vi "vew -- array interpolate.vi"() -> ()   [LabVIEW 2010]
uses:
  Q -- check range -- i -- real.vi
  Q - not nan -- real.vi
  <vilib>/gmath/function.llb/Binomial Coefficient.vi
panel:
  in  "N":i32=100
  in  "freq max":dbl=300.0
  in  "freq min":dbl=10.0
  out "Plot: phase around center":cluster{dbl[], dbl[]}[](graph)=[{array[1389 elements], array[1389 elements]}, {[3015.8552146531347, 3016.2383756063605, 3016.6215365595863], [1.7830935388456814, 3.353889865640578, 4.924686192435475]}, {array[1389 elements], array[1389 elements]}]
  in  "all Voltage":dbl[](array[numeric])=[0.1, 0.5, 0.2, 0.9]
  in  "all tempearure":dbl[](array[numeric])=[10.0, 70.0, 150.0, 300.0]
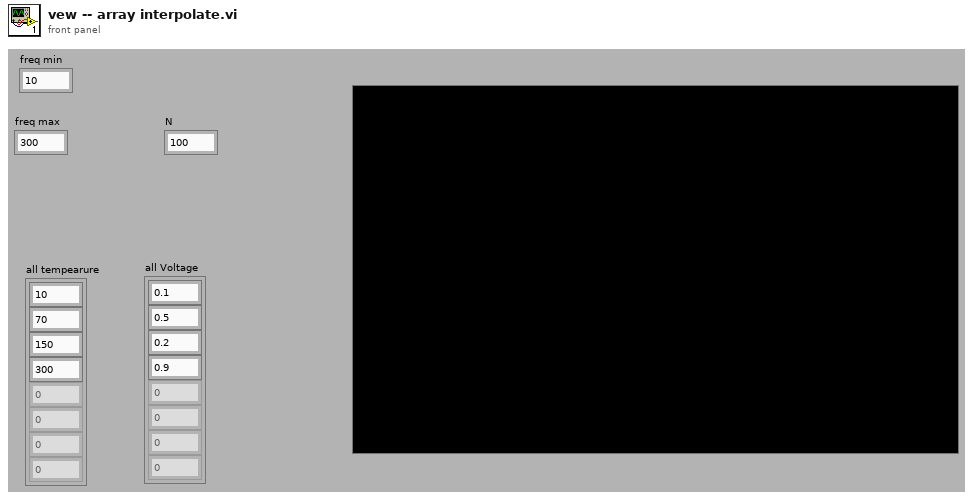
[diagram p1: front panel]
types:
  T1 = cluster{"all tempearure":dbl[], "all Voltage":dbl[]}
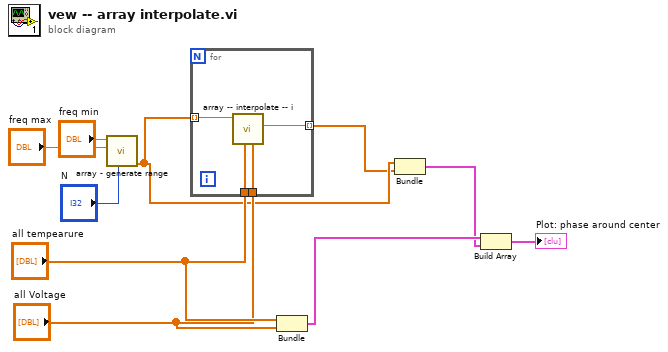
[diagram p0: block diagram]
diagram:
  n1 = call "array - generate range.vi"("N"="N", "freq max"="freq max", "freq min"="freq min") -> ("Array"=w4:dbl[])  [unwired: 8 in]
  n2 = for {
    tunnel: "all tempearure" -> [w14]
    tunnel: "all Voltage" -> [w13]
    tunnel: w4 -> [w12] mode=indexing
    tunnel: [w11] -> w3 mode=indexing
    n3 = call "array -- interpolate -- i.vi"("all Voltage"=w13, "all tempearure"=w14, "temperature (K)"=w12) -> ("V out"=w11:dbl)  [unwired: 8 in]
  }
  n4 = Bundle("all tempearure"="all tempearure", "all Voltage"="all Voltage") -> (w8:T1)  [unwired: 1 in]
  n5 = Bundle("Array"=w4, w3) -> (w2:cluster{"Array":dbl[], dbl[]})  [unwired: 1 in]
  n6 = Build Array(w8, w2) -> (→"Plot: phase around center":cluster{"Array":dbl[], "all Voltage":dbl[]}[])
